vi "Query Signal Lists.vi"(8 "error in (no error)":errorcluster, 11 "CAN Configurations in":T1[](array[typedef]) {"Sample Rate (Hz)" format="%#_13g"}) -> (0 "error out":errorcluster, 2 "Signal Units":string[](array[string]), 3 "Signal Names":string[](array[string]))   [LabVIEW 2021, in "XNET-CAN-Signal-Logger.lvlib"]
uses:
  XNET-CAN-Signal-Logger.lvlib
  Typedef/Def-CAN Port Configuration.ctl
  SubVIs/Global Variables.vi
  <resource>/objmgr/xnet.rc
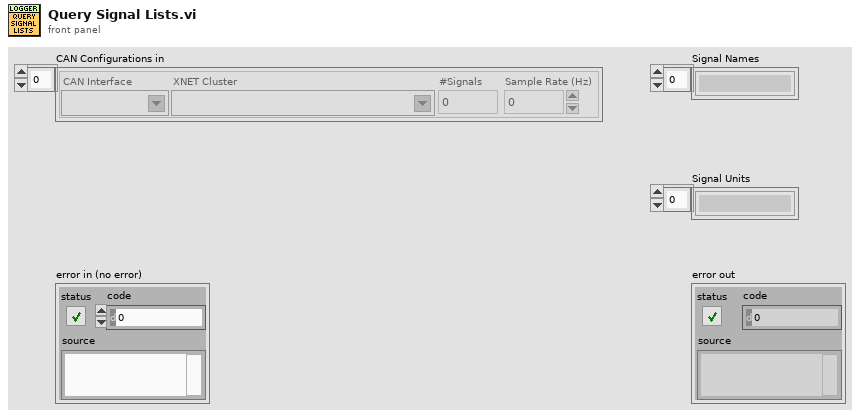
[diagram p1: front panel]
types:
  T1 = typedef "XNET-CAN-Signal-Logger.lvlib/Def-CAN Port Configuration.ctl" = cluster{"CAN Interface":refnum<k21>, "XNET Cluster":refnum<k21>, "#Signals":i32, "Sample Rate (Hz)":dbl}
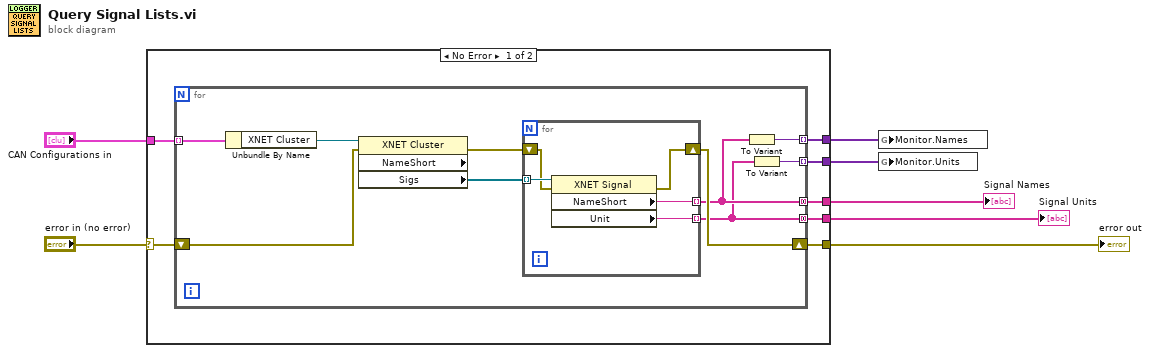
[diagram p0: block diagram]
diagram:
  n1 = case shown="No Error" "error in (no error)" {
    selector: "error in (no error)" -> [w11 w30]
    tunnel: [w14 _] -> w7
    tunnel: "CAN Configurations in" -> [w13 _]
    tunnel: [w12 _] -> w5
    tunnel: [w10 w30] -> w3
    tunnel: [w9 _] -> w2
    tunnel: [w8 _] -> w1
    frame No Error {
      n2 = for {
        tunnel: [w18] -> w14 mode=concatenating
        tunnel: w13 -> [w23] mode=indexing
        tunnel: [w16] -> w12 mode=concatenating
        shift-right: [w19] -> w10
        shift-left: w11 -> [w21]
        tunnel: [w17] -> w9 mode=indexing
        tunnel: [w15] -> w8 mode=indexing
        n3 = Unbundle By Name(w23) -> ("XNET Cluster"=w22:refnum<k21>)
        n4 = property class="XNET Cluster" props=["NameShort", "Sigs"](reference=w22, error in=w21) -> (error out=w20:errorcluster, "Sigs"=w24:refnum<k21>[])  [unwired: 2 out]
        n5 = for {
          tunnel: w24 -> [w29] mode=indexing
          tunnel: [w28] -> w18 mode=indexing
          tunnel: [w27] -> w16 mode=indexing
          shift-right: [w25] -> w19
          shift-left: w20 -> [w26]
          n6 = property class="XNET Signal"(reference=w29, error in=w26) -> (error out=w25:errorcluster, "NameShort"=w28:string, "Unit"=w27:string)  [unwired: 1 out]
        }
        n7 = To Variant(anything=w18) -> (Variant=w17:variant)
        n8 = To Variant(anything=w16) -> (Variant=w15:variant)
      }
    }
    frame Error {
    }
  }
  "Signal Names" <- w7
  "Signal Units" <- w5
  "error out" <- w3
  n9 = global write "Global Variables.vi" "Monitor.Names"(w2) -> ()
  n10 = global write "Global Variables.vi" "Monitor.Units"(w1) -> ()
